vi "Find intersection rows and columns.vi"(11 "Page intersection array":bool[][](array[boolean])) -> (2 "Columns":i32[](array[numeric]), 3 "Rows":i32[](array[numeric]))   [LabVIEW 2023]
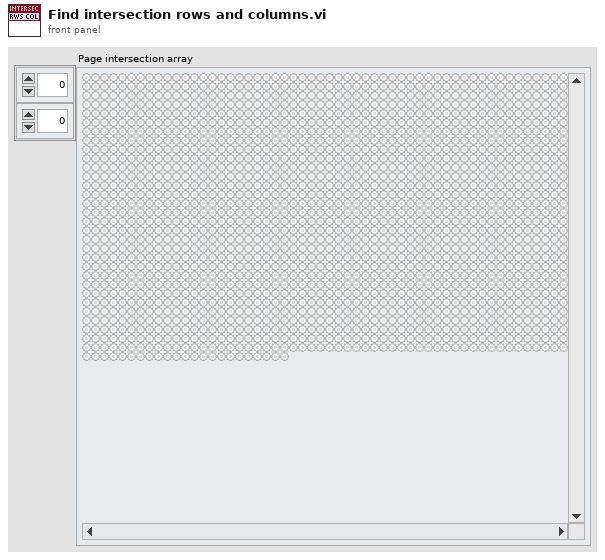
[diagram p1: front panel]
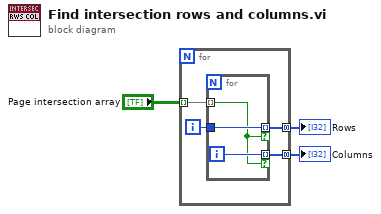
[diagram p0: block diagram]
diagram:
  n1 = for {
    tunnel: "Page intersection array" -> [w7] mode=indexing
    tunnel: [w5] -> w2 mode=concatenating
    tunnel: [w4] -> w1 mode=concatenating
    i -> [w6]
    n2 = for {
      tunnel: w7 -> [w8] mode=indexing
      tunnel: w6 -> [w9]
      tunnel: [w10] -> w4 mode=indexing if=w8
      tunnel: [w9] -> w5 mode=indexing if=w8
      i -> [w10]
    }
  }
  "Rows" <- w2
  "Columns" <- w1
